vi "Write Base Actor.vi"(10 "Base Actor":T1, 11 "TEMPLATE Actor in":refnum<class "TEMPLATE Actor.lvclass">) -> (3 "TEMPLATE Actor out":refnum<class "TEMPLATE Actor.lvclass">)   [LabVIEW 2020, in "_Template.lvlib" / "Templates.lvlib" / "TEMPLATE jettl Actor.lvlib" / "TEMPLATE Actor.lvlib" / "TEMPLATE Actor.lvclass"]
uses:
  TEMPLATE Actor.lvclass
  TEMPLATE Actor.lvclass/TEMPLATE Actor.ctl
  jettl/jettl/Actor/Actor.lvclass
  jettl/jettl/Lifetime.ctl
  jettl/jettl/jettl.lvlib
  jettl/jettl/Base Actor.ctl
panel:
  # "This front panel should not be manipulated."
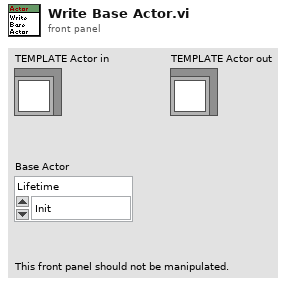
[diagram p1: front panel]
types:
  T1 = typedef "jettl.lvlib/Base Actor.ctl" = cluster{"Lifetime":T2}
  T2 = typedef "jettl.lvlib/Lifetime.ctl" = enum16{"Init", "Spawn", "Setup", "Teardown Before Running", "Running", "Stop Called", "Stopping With Children", "Stopping Without Children", "Teardown After Running", "Stopped"}
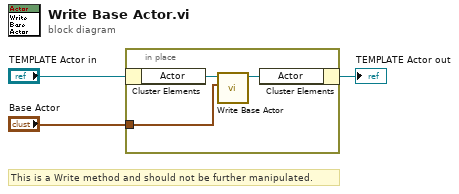
[diagram p0: block diagram]
diagram:
  # "This is a Write method and should not be further manipulated."
  n1 = in-place {
    in-place-border: "Base Actor" -> [w4]
    n2 = in-place-cluster #1("TEMPLATE Actor in") -> ("Actor"=w6:refnum<class "Actor.lvclass">)
    n3 = call-dynamic "Write Base Actor.vi"("Base Actor"=w4, "Actor in"=w6) -> ("Actor out"=w5:refnum<class "Actor.lvclass">)  [unwired: 9 in]
    n4 = in-place-cluster #1("Actor"=w5) -> (→"TEMPLATE Actor out":refnum<class "TEMPLATE Actor.lvclass">)
  }
